vi "test write api.vi"() -> ()   [LabVIEW 2019]
uses:
  <vilib>/httpClient/POSTBuffer.vi
  <vilib>/httpClient/LabVIEWHTTPClient.lvlib
panel:
  out "before substring":string
  out "body":string
  out "JSON string":string
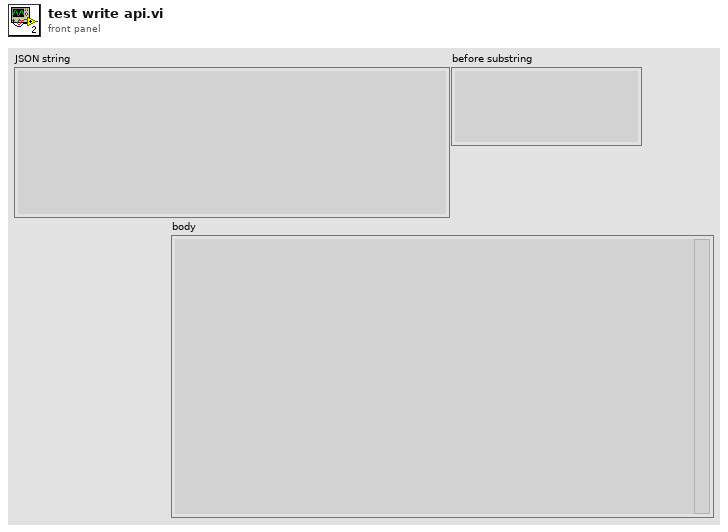
[diagram p1: front panel]
types:
  T1 = cluster{"testname":string, "jobno":string, "jobdesc":string, "sampleid":string, "date":string}
  T2 = cluster{"timestamp":string, "elapsetime":string, "testname":string, "testtype":u16, "data":string[]}
  T3 = typedef "LabVIEWHTTPClient.lvlib/ClientHandle.ctl" = refnum<k1>
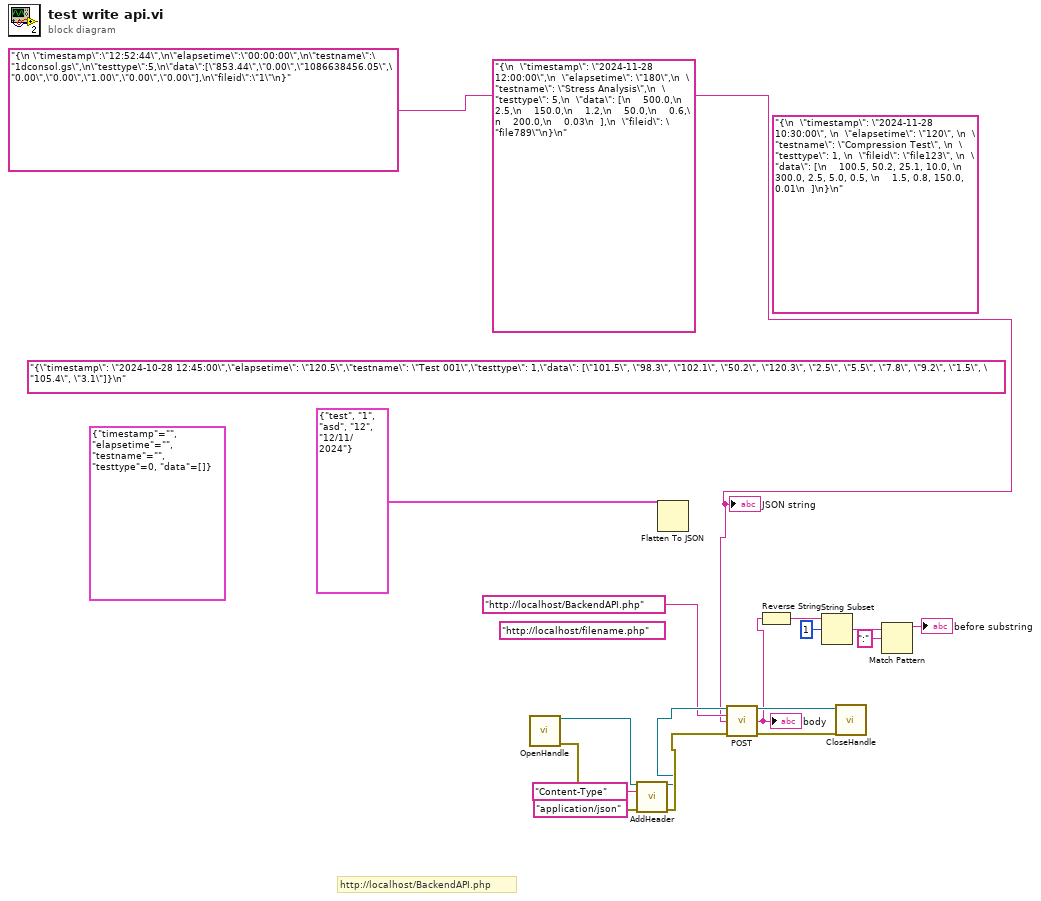
[diagram p0: block diagram]
diagram:
  (unwired) "{\n  \"timestamp\": \"2024-11-28 12:00:00\",\n  \"elapsetime\": \"180\",\n  \"testname\": \"Stress Analysis\",\n  \"testtype\": 5,\n  \"data\": [\n    500.0,\n    2.5,\n    150.0,\n    1.2,\n    50.0,\n    0.6,\n    200.0,\n    0.03\n  ],\n  \"fileid\": \"file789\"\n}\n"
  w1 = "{\n \"timestamp\":\"12:52:44\",\n\"elapsetime\":\"00:00:00\",\n\"testname\":\"1dconsol.gs\",\n\"testtype\":5,\n\"data\":[\"853.44\",\"0.00\",\"1086638456.05\",\"0.00\",\"0.00\",\"1.00\",\"0.00\",\"0.00\"],\n\"fileid\":\"1\"\n}"
  (unwired) "http://localhost/filename.php" ("url")
  (unwired) "{\n  \"timestamp\": \"2024-11-28 10:30:00\", \n  \"elapsetime\": \"120\", \n  \"testname\": \"Compression Test\", \n  \"testtype\": 1, \n  \"fileid\": \"file123\", \n  \"data\": [\n    100.5, 50.2, 25.1, 10.0, \n    300.0, 2.5, 5.0, 0.5, \n    1.5, 0.8, 150.0, 0.01\n  ]\n}\n"
  (unwired) T2 {"timestamp"="", "elapsetime"="", "testname"="", "testtype"=0, "data"=[]}
  (unwired) "{\"timestamp\": \"2024-10-28 12:45:00\",\"elapsetime\": \"120.5\",\"testname\": \"Test 001\",\"testtype\": 1,\"data\": [\"101.5\", \"98.3\", \"102.1\", \"50.2\", \"120.3\", \"2.5\", \"5.5\", \"7.8\", \"9.2\", \"1.5\", \"105.4\", \"3.1\"]}\n"
  # "http://localhost/BackendAPI.php"
  n1 = call <vilib>:"OpenHandle.vi"() -> ("client handle out"=w12:T3, "error out"=w14:errorcluster)  [unwired: 14 in]
  n2 = call <vilib>:"AddHeader.vi"("client handle"=w12, "header"="Content-Type", "value"="application/json", "error in (no error)"=w14) -> ("client handle out"=w11:T3, "error out"=w13:errorcluster)  [unwired: 10 in]
  n3 = Flatten To JSON(anything=T1 {"testname"="test", "jobno"="1", "jobdesc"="asd", "sampleid"="12", "date"="12/11/2024"}) -> ()  [unwired: 2 in, 2 out]
  n4 = call-poly <vilib>:"POST.vi"("client handle"=w11, "url"="http://localhost/BackendAPI.php", "buffer"=w1, "error in (no error)"=w13) -> ("client handle out"=w15:T3, "body"=w4:string, "error out"=w16:errorcluster)  [unwired: 8 in, 1 out]
  "body" <- w4
  n5 = Reverse String(1:w4) -> (0:w7:string)
  n6 = String Subset(string=w7, offset (0)=1) -> (substring=w6:string)  [unwired: 1 in]
  n7 = call <vilib>:"CloseHandle.vi"("client handle"=w15, "error in (no error)"=w16) -> ()  [unwired: 13 in, 1 out]
  n8 = Match Pattern(string=w6, regular expression=":") -> (before substring=→"before substring":string)  [unwired: 1 in, 3 out]
  "JSON string" <- w1
